vi "Flywheel_Globals.vi"() -> ()   [LabVIEW 2019]
uses:
  Subsystems/Flywheel/Flywheel_Cluster.ctl
  Subsystems/Flywheel/Flywheel_States.ctl
  Utility VIs/Basic_Motor_Modes.ctl
panel:
  in  "Flywheel_Table":dbl[][](array[numeric])
  in  "Flywheel_Output":dbl
  in  "Motor_Mode":T1
  out "Spun_Up":bool
  in  "Flywheel_Execute_Notifier":refnum<notifier>
  in  "Flywheel_Set_Notifier":refnum<notifier>
  in  "Flywheel_Set_Ref":string="Flywheel_Set_Ref"
  in  "Flywheel_Execute_Ref":string="Flywheel_Execute_Ref"
  in  "Flywheel_Left":string="Flywheel_Left"
  in  "Flywheel_Right":string="Flywheel_Right"
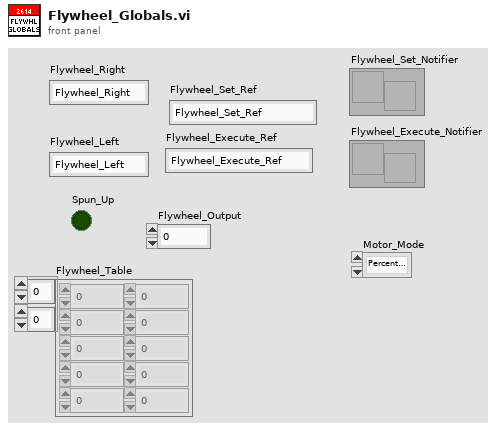
[diagram p1: front panel]
types:
  T1 = typedef "Basic_Motor_Modes.ctl" = enum16{"Percent_Voltage", "Speed_Control", "Position_Control", "Current"}
diagram:
